vi "PRM1Z8_setPower.vi"(8 "error in (no error)":errorcluster, 10 "Target Power":dbl, 11 "reference":refnum<k24>) -> (0 "error out":errorcluster, 3 "reference out":refnum<k24>)   [LabVIEW 2018, in "Laser Quantum.lvlib"]
uses:
  Laser Quantum.lvlib
  C:/Program Files/Thorlabs/Kinesis/ThorLabs.MotionControl.KCube.DCServoCLI.dll
  Program Files/Thorlabs/Kinesis/ThorLabs.MotionControl.KCube.DCServoCLI.dll
panel:
  out "output angle":dbl
  in  "zero angle":dbl
  in  "max power":dbl=2520.0
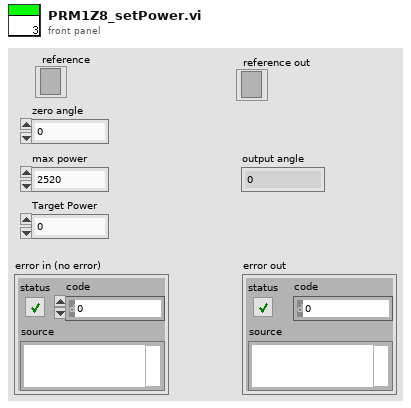
[diagram p1: front panel]
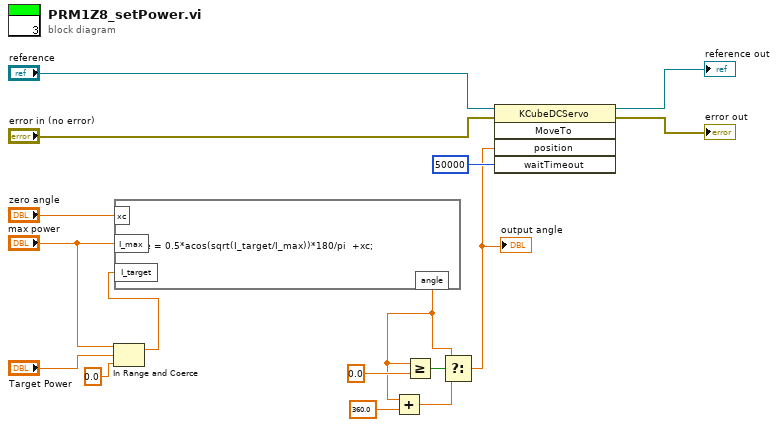
[diagram p0: block diagram]
diagram:
  n1 = In Range and Coerce(upper limit="max power", x="Target Power", lower limit=0.0) -> (coerced(x)=w5:dbl)  [unwired: 1 out]
  n2 = formula code="angle = 0.5*acos(sqrt(I_target/I_max))*180/pi  +xc;"("I_target"=w5, "I_max"="max power", "xc"="zero angle") -> ("angle"=w9:dbl)
  n3 = Add(x=w9, y=360.0) -> (x+y=w12:dbl)
  n4 = Greater Or Equal?(x=w9, y=0.0) -> (x >= y?=w8:bool)
  n5 = Select(t=w9, s=w8, f=w12) -> (s? t:f=w13:dbl)
  "output angle" <- w13
  n6 = invoke class="KCubeDCServo" method="MoveTo"(reference="reference", error in="error in (no error)", "position"=w13, "waitTimeout"=50000) -> (reference out=→"reference out":refnum<k24>, error out=→"error out":errorcluster)  [unwired: 1 in, 3 out]
